vi "Fluke Molbox 1 Plus Acquire Average Flow Cycle Results.vi"(0 "VISA resource name":refnum<visa-resource-name>, 5 "Period (500)":i32=500 min=4 max=999, 7 "Enable MFC (Enable)":bool=TRUE, 9 "MFC Channel (Channel 1)":i32(ring)=1 items=["Channel 1"=1, "Channel 2"=2, "Channel 3"=3, "Channel 4"=4, "Channel 5"=5], 12 "MFC Mode (Voltage)":u16(ring) items=["Voltage", "Current"]) -> (6 "Flow Stability":bool, 8 "Flow Measurements":T2, 10 "MFC Voltage or Current":dbl, 14 "MFC Voltage or Current Average":dbl)   [LabVIEW 2023]
doc: "Completes an average flow cycle of a user generated period. Returns results from the averaging flow cycle that can only be used following an averaging flow cycle."
uses:
  Fluke Molbox 1 Plus.lvlib
panel:
  in  "Serial Configuration":T1={"Baud Rate"=9600, "Parity"=0, "Data Bits"=7, "Stop Bits"=10} {"Stop Bits" items=["1"=10, "2"=20]; "Data Bits" items=["7"=7, "8"=8]; "Parity" items=["None", "Odd", "Even"]; "Baud Rate" items=["300"=300, "600"=600, "1200"=1200, "2400"=2400, "4800"=4800, "9600"=9600, "19200"=19200]}
  # "(c) 2012 National Instruments.  ALL RIGHTS RESERVED."
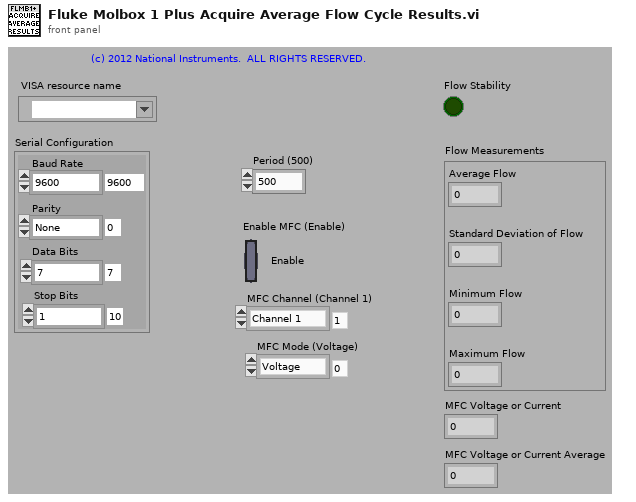
[diagram p1: front panel]
types:
  T1 = cluster{"Baud Rate":u32, "Parity":u16, "Data Bits":u16, "Stop Bits":u16}
  T2 = cluster{"Maximum Flow":dbl, "Minimum Flow":dbl, "Standard Deviation of Flow":dbl, "Average Flow":dbl}
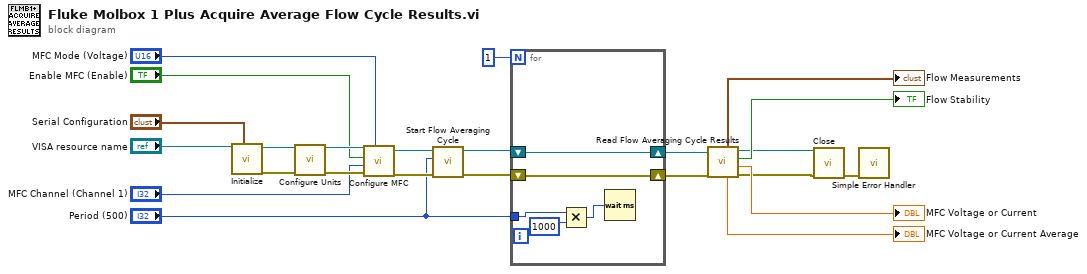
[diagram p0: block diagram]
diagram:
  n1 = call "Initialize.vi"("Serial Configuration"="Serial Configuration", "VISA resource name"="VISA resource name") -> ("error out"=w22:errorcluster, "VISA resource name out"=w23:refnum<visa-resource-name>)  [unwired: 8 in]
  n2 = call "Configure Units.vi"("VISA resource name"=w23, "error in (no error)"=w22) -> ("VISA resource name out"=w21:refnum<visa-resource-name>, "error out"=w20:errorcluster)  [unwired: 12 in]
  n3 = call "Configure MFC.vi"("MFC Mode (0: Voltage)"="MFC Mode (Voltage)", "error in (no error)"=w20, "MFC Channel (1: Channel 1)"="MFC Channel (Channel 1)", "Enable MFC (Enable)"="Enable MFC (Enable)", "VISA resource name"=w21) -> ("error out"=w15:errorcluster, "VISA resource name out"=w16:refnum<visa-resource-name>)  [unwired: 5 in]
  n4 = call "Start Flow Averaging Cycle.vi"("error in (no error)"=w15, "Period (500)"="Period (500)", "VISA resource name"=w16) -> ("error out"=w13:errorcluster, "VISA resource name out"=w14:refnum<visa-resource-name>)  [unwired: 7 in]
  n5 = for {
    N: 1 -> [_]
    shift-right: [w26] -> w11
    shift-left: w13 -> [w26]
    shift-right: [w25] -> w12
    shift-left: w14 -> [w25]
    tunnel: "Period (500)" -> [w28]
    n6 = Multiply(x=w28, y=1000) -> (x*y=w29:i32)
    n7 = Wait (ms)(milliseconds to wait=w29) -> ()  [unwired: 1 out]
  }
  n8 = call "Read Flow Averaging Cycle Results.vi"("error in (no error)"=w11, "VISA resource name"=w12) -> ("error out"=w2:errorcluster, "MFC Voltage or Current"=→"MFC Voltage or Current":dbl, "Flow Stability"=→"Flow Stability":bool, "VISA resource name out"=w1:refnum<visa-resource-name>, "MFC Voltage or Current Average"=→"MFC Voltage or Current Average":dbl, "Flow Measurements"=→"Flow Measurements":T2)  [unwired: 4 in]
  n9 = call "Close.vi"("error in (no error)"=w2, "VISA resource name"=w1) -> ("error out"=w4:errorcluster)  [unwired: 9 in]
  n10 = call <vilib>:"Simple Error Handler.vi"("error in (no error)"=w4) -> ()  [unwired: 4 in, 5 out]
